vi "intakeRoller.vi"() -> ()   [LabVIEW 2018]
uses:
  intakeRoller.ctl
panel:
  in  "speedControl":dbl=0.7
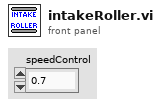
[diagram p1: front panel]
types:
  T1 = typedef "intakeRoller.ctl" = enum16{"off", "intake", "outtake"}
  T2 = typedef "WPI_MotorControlDeviceRef.ctl" = cluster{"DeviceStatus":errorcluster, "Type":T3, "PWM":cluster{"PWM Channel":T4, "DeadBand":T5}, "CAN":cluster{"Device Number":u8, "SetOutput VI Ref":variant, "GetOutput VI Ref":variant, "Enable VI Ref":variant, "Disable VI Ref":variant, "Data":variant}, "Invert":bool, "DIO PWM":cluster{"PWM \"Enable\" Channel":T4, "DIOChannel":T6, "PWM Rate":dbl}}
  T3 = typedef "WPI_MotorControlType.ctl" = enum16{"PWM", "CAN", "DIO PWM"}
  T4 = typedef "FPGA_DIOPWMChannel.ctl" = enum8{"PWM 0", "PWM 1", "PWM 2", "PWM 3", "PWM 4", "PWM 5", "PWM 6", "PWM 7", "PWM 8", "PWM 9", "PWM MXP 0", "PWM MXP 1", "PWM MXP 2", "PWM MXP 3", "PWM MXP 4", "PWM MXP 5", "PWM MXP 6", "PWM MXP 7", "PWM MXP 8", "PWM MXP 9", "Invalid"}
  T5 = typedef "WPI_PWMDeadband.ctl" = cluster{"Name":string, "maxPositivePwm":i32, "minPositivePwm":i32, "centerPwm":i32, "maxNegativePwm":i32, "minNegativePwm":i32, "angularRange":u16}
  T6 = typedef "FPGA_DIOChannel.ctl" = enum8{"DIO 0", "DIO 1", "DIO 2", "DIO 3", "DIO 4", "DIO 5", "DIO 6", "DIO 7", "DIO 8", "DIO 9", "DIO MXP 0", "DIO MXP 1", "DIO MXP 2", "DIO MXP 3", "DIO MXP 4", "DIO MXP 5", "DIO MXP 6", "DIO MXP 7", "DIO MXP 8", "DIO MXP 9", "DIO MXP 10", "DIO MXP 11", "DIO MXP 12", "DIO MXP 13", "DIO MXP 14", "DIO MXP 15", "SPI Port CS1", "SPI Port CS2", "SPI Port CS3", "SPI Port MISO", "SPI Port MOSI", "Invalid"}
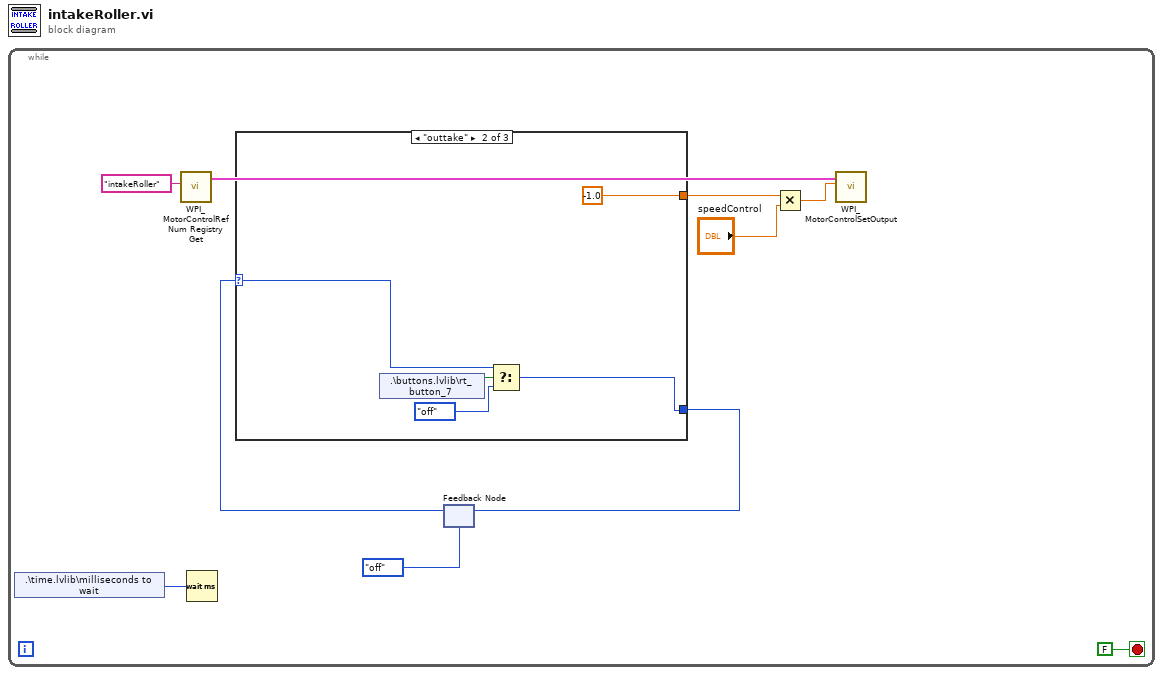
[diagram p0: block diagram]
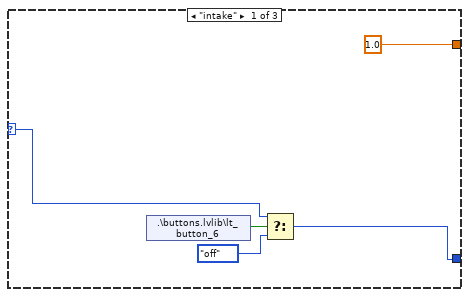
[diagram p2: hidden frame]
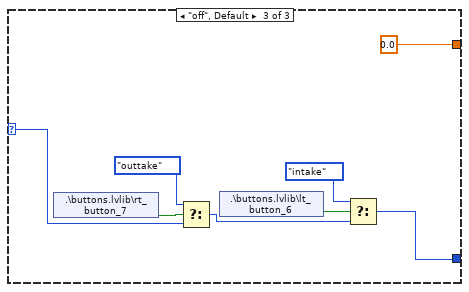
[diagram p3: hidden frame]
diagram:
  n1 = while {
    stop <- FALSE stop-if-true
    n2 = shared-variable ".\\time.lvlib\\milliseconds to wait"() -> (w5:u32)  [unwired: 1 in, 1 out]
    n3 = call <vilib>:"WPI_MotorControlRefNum Registry Get.vi"("refnum name"="intakeRoller") -> ("MotorControlDevRef"=w9:T2)  [unwired: 9 in, 1 out]
    n4 = Wait (ms)(milliseconds to wait=w5) -> ()  [unwired: 1 out]
    n5 = feedback #1(intakeRoller."off") -> (w6:T1)
    n6 = case shown="\"outtake\"" w6 {
      selector: w6 -> [w13 w19 w28]
      tunnel: [w14 w17 w26] -> w8
      tunnel: [1.0 ("Output") -1.0 ("Output") 0.0 ("Output")] -> w3
      frame "intake" {
        n7 = shared-variable ".\\buttons.lvlib\\lt_button_6"() -> (w15:bool)  [unwired: 1 in, 1 out]
        n8 = Select(t=w13, s=w15, f=intakeRoller."off") -> (s? t:f=w14:T1)
      }
      frame "outtake" {
        n9 = shared-variable ".\\buttons.lvlib\\rt_button_7"() -> (w18:bool)  [unwired: 1 in, 1 out]
        n10 = Select(t=w19, s=w18, f=intakeRoller."off") -> (s? t:f=w17:T1)
      }
      frame "off", Default {
        n11 = shared-variable ".\\buttons.lvlib\\rt_button_7"() -> (w25:bool)  [unwired: 1 in, 1 out]
        n12 = Select(t=intakeRoller."outtake", s=w25, f=w28) -> (s? t:f=w27:T1)
        n13 = shared-variable ".\\buttons.lvlib\\lt_button_6"() -> (w24:bool)  [unwired: 1 in, 1 out]
        n14 = Select(t=intakeRoller."intake", s=w24, f=w27) -> (s? t:f=w26:T1)
      }
    }
    n15 = feedback-in #1(w8) -> ()
    n16 = Multiply(x=w3, y="speedControl") -> (x*y=w2:dbl)
    n17 = call <vilib>:"WPI_MotorControlSetOutput.vi"("Output"=w2, "MotorControlDevRef"=w9) -> ()  [unwired: 7 in, 3 out]
  }
